vi "NI VeriStand - Set Custom Device Drivers.vi"(7 "Execution mode":T5, 8 "error in (no error)":errorcluster, 9 "Version":string, 10 "Driver VI":T1[](array[typedef]), 11 "Device Ref in":T6 format="%.0x") -> (0 "error out":errorcluster, 3 "Device Ref out":T6 format="%.0x")   [LabVIEW 2020, in "Custom Device API.lvlib"]
doc: "Sets the RT Driver VI(s) for a custom device. Use this VI to associate multiple driver VIs with a custom device or to programmatically change the driver VI for a custom device. Multiple driver VIs can be necessary if the device runs on multiple targets with different operating systems, or if the device runs in different execution modes (for example, Inline HW Interface and Asynchronous)."
uses:
  <vilib>/NI VeriStand/Custom Device API/Custom Device API.lvlib
  <vilib>/NI VeriStand/Custom Device API/Custom Device Item Ref.ctl
  <vilib>/NI VeriStand/Custom Device API/Custom Device Execution Mode.ctl
  <vilib>/NI VeriStand/Custom Device API/Custom Device Path Data.ctl
  <vilib>/NI VeriStand/Custom Device API/Custom Device Supported Target.ctl
  <vilib>/NI VeriStand/Custom Device API/Path Specification.ctl
  <vilib>/NI VeriStand/Custom Device API/Path Type.ctl
  9351174d-25e8-4c9c-b819-99678f856bef.vi
  <vilib>/NI VeriStand/Custom Device API/Custom Device Offline Path.vi
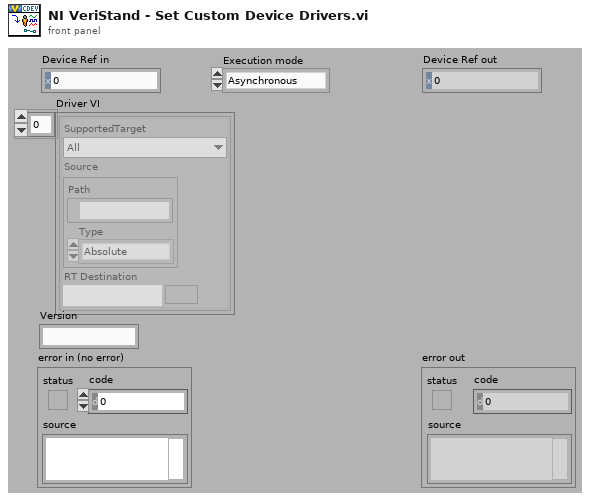
[diagram p1: front panel]
types:
  T1 = typedef "Custom Device API.lvlib/Custom Device Path Data.ctl" = cluster{"SupportedTarget":T2, "Source":T3, "RT Destination":path}
  T2 = typedef "Custom Device API.lvlib/Custom Device Supported Target.ctl" = enum16{"All", "PharLap", "VxWorks", "Windows", "Linux_32_ARM", "Linux_x64", "PharLap & Windows", "PharLap & VxWorks", "VxWorks & Windows"}
  T3 = typedef "Custom Device API.lvlib/Path Specification.ctl" = cluster{"Path":path, "Type":T4}
  T4 = typedef "Custom Device API.lvlib/Path Type.ctl" = enum16{"Absolute", "To Base", "To Common Data Dir", "To Application Data Dir"}
  T5 = typedef "Custom Device API.lvlib/Custom Device Execution Mode.ctl" = enum16{"Asynchronous", "Inline HW Interface", "Inline Model Interface", "Inline Timing and Sync", "Asynchronous Timing and Sync"}
  T6 = typedef "Custom Device API.lvlib/Custom Device Item Ref.ctl" = u64
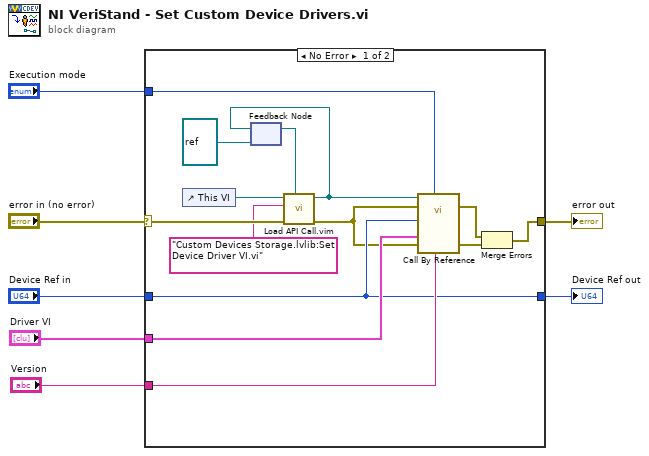
[diagram p0: block diagram]
diagram:
  n1 = case shown="No Error" "error in (no error)" {
    selector: "error in (no error)" -> [w13 w23]
    tunnel: "Execution mode" -> [w20 _]
    tunnel: "Device Ref in" -> [w16 w22]
    tunnel: [w19 w23] -> w5
    tunnel: [w16 w22] -> w4
    tunnel: "Driver VI" -> [w18 _]
    tunnel: "Version" -> [w17 _]
    frame No Error {
      n2 = control-ref of="This VI"() -> (w14:refnum<vi>)
      n3 = feedback #1(refnum<vi> refnum ("type specifier VI Refnum (for type only)")) -> (w15:refnum<vi>)
      n4 = call "Load API Call.vim"("VI reference in"=w15, "error in (no error)"=w13, "VI qualified name"="Custom Devices Storage.lvlib:Set Device Driver VI.vi", "Caller VI ref"=w14) -> ("error out"=w12:errorcluster, "VI reference"=w11:refnum<vi>)  [unwired: 6 in]
      n5 = feedback-in #1(w11) -> ()
      n6 = call-by-ref "?"(reference=w11, error in=w12, "Version"=w17, "Execution mode"=w20, 8:"error in (no error)"=w12, "Driver VI"=w18, "Device Ref in"=w16) -> (error out=w8:errorcluster, 0:"error out"=w21:errorcluster)  [unwired: 5 in, 2 out]
      n7 = Merge Errors(w8, w21) -> (w19:errorcluster)
    }
    frame Error {
    }
  }
  "Device Ref out" <- w4
  "error out" <- w5
